vi "Display Message.vi"(8 "error in (no error)":errorcluster, 10 "Message":string, 11 "Demo1 in":refnum<class "Demo1.lvclass">) -> (0 "error out":errorcluster, 3 "Demo1 out":refnum<class "Demo1.lvclass">)   [LabVIEW 2020, in "Demo1.lvlib" / "Demo1.lvclass"]
uses:
  Demo1.lvclass
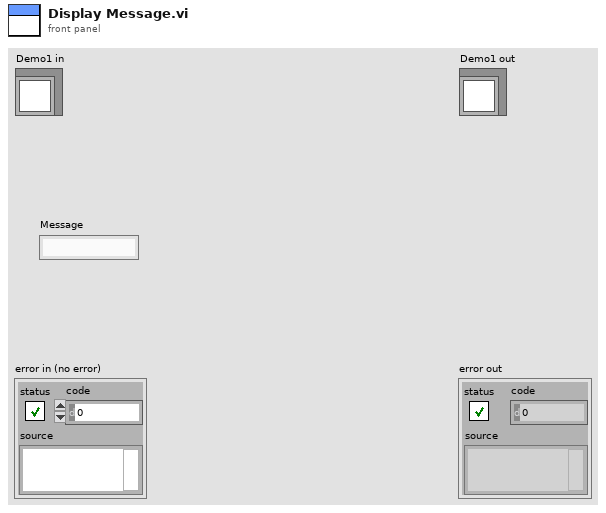
[diagram p1: front panel]
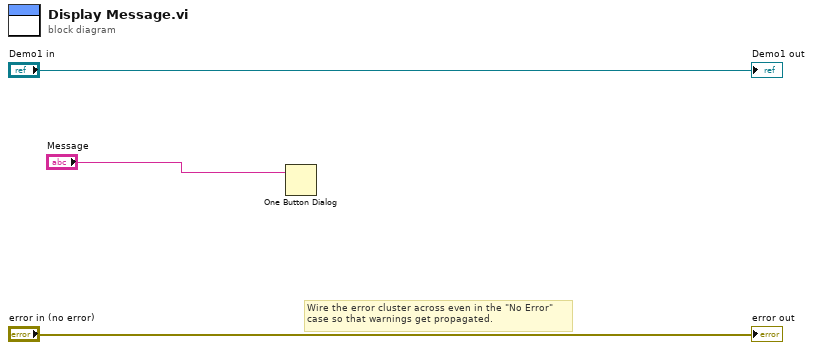
[diagram p0: block diagram]
diagram:
  # "Wire the error cluster across even in the \"No Error\"\ncase so that warnings get propagated."
  n1 = One Button Dialog(message="Message") -> ()  [unwired: 1 in, 1 out]
  "error out" <- "error in (no error)"
  "Demo1 out" <- "Demo1 in"
